vi "1.TCP客户端接收JPEG图片流.vi"() -> ()   [LabVIEW 2018]
panel:
  in  "停止":bool
  out "new picture":picture
  out "接收字符串":string
  out "开始flag":bool=TRUE
  in  "?":string="8088"
  in  "地址输入端":string="192.168.1.30"
  # "地   址："
  # "端口号："
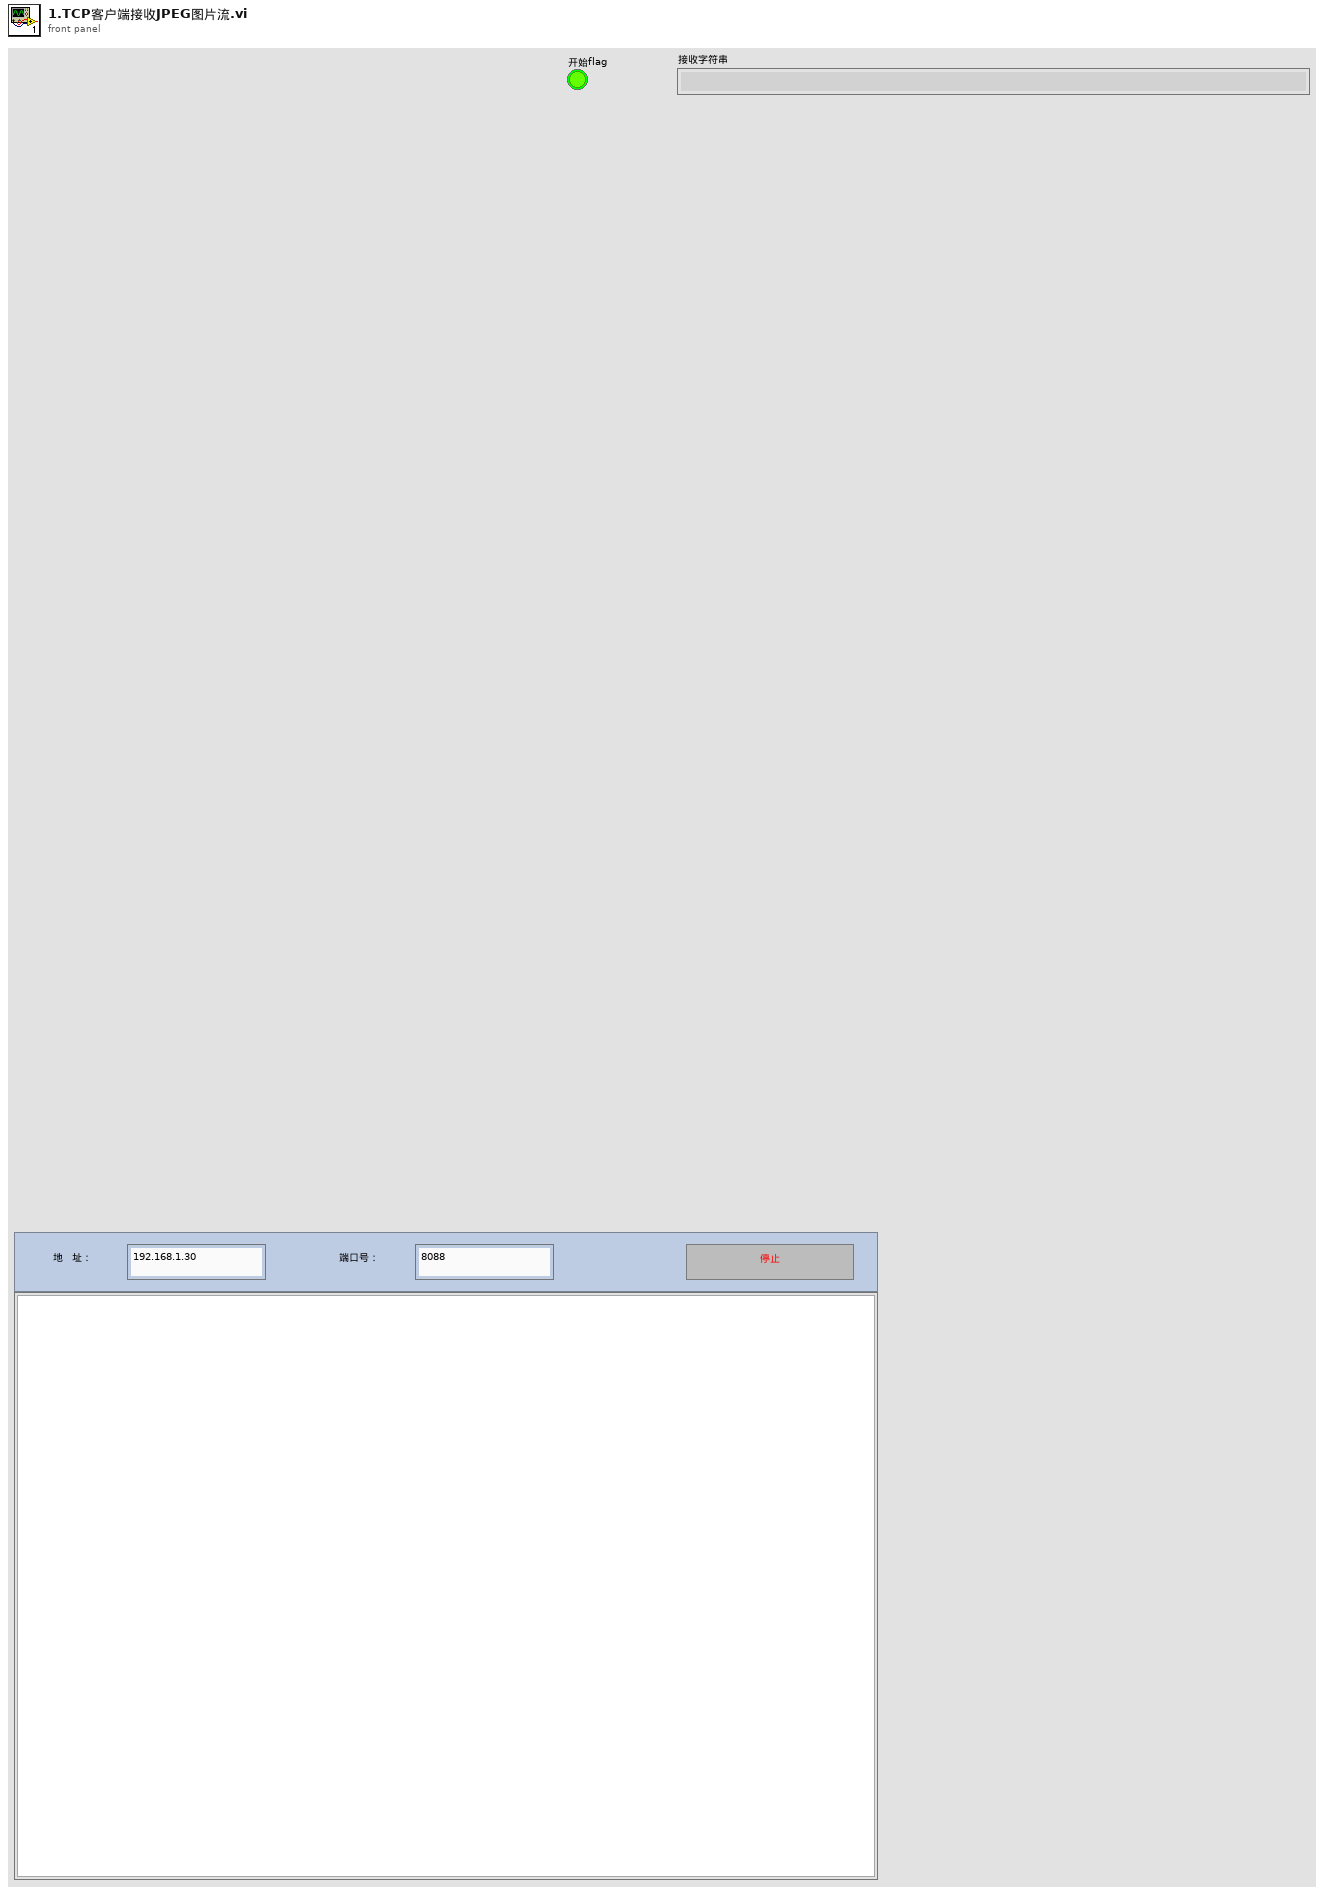
[diagram p1: front panel]
types:
  T1 = enum16{"open", "replace", "create", "open or create", "replace or create", "replace or create with confirmation"}
  T2 = typedef "imagedata.ctl" = cluster{"image type":i32, "image depth":i32, "image":u8[], "mask":u8[], "colors":u32[], "Rectangle":cluster{"left":i16, "top":i16, "right":i16, "bottom":i16}}
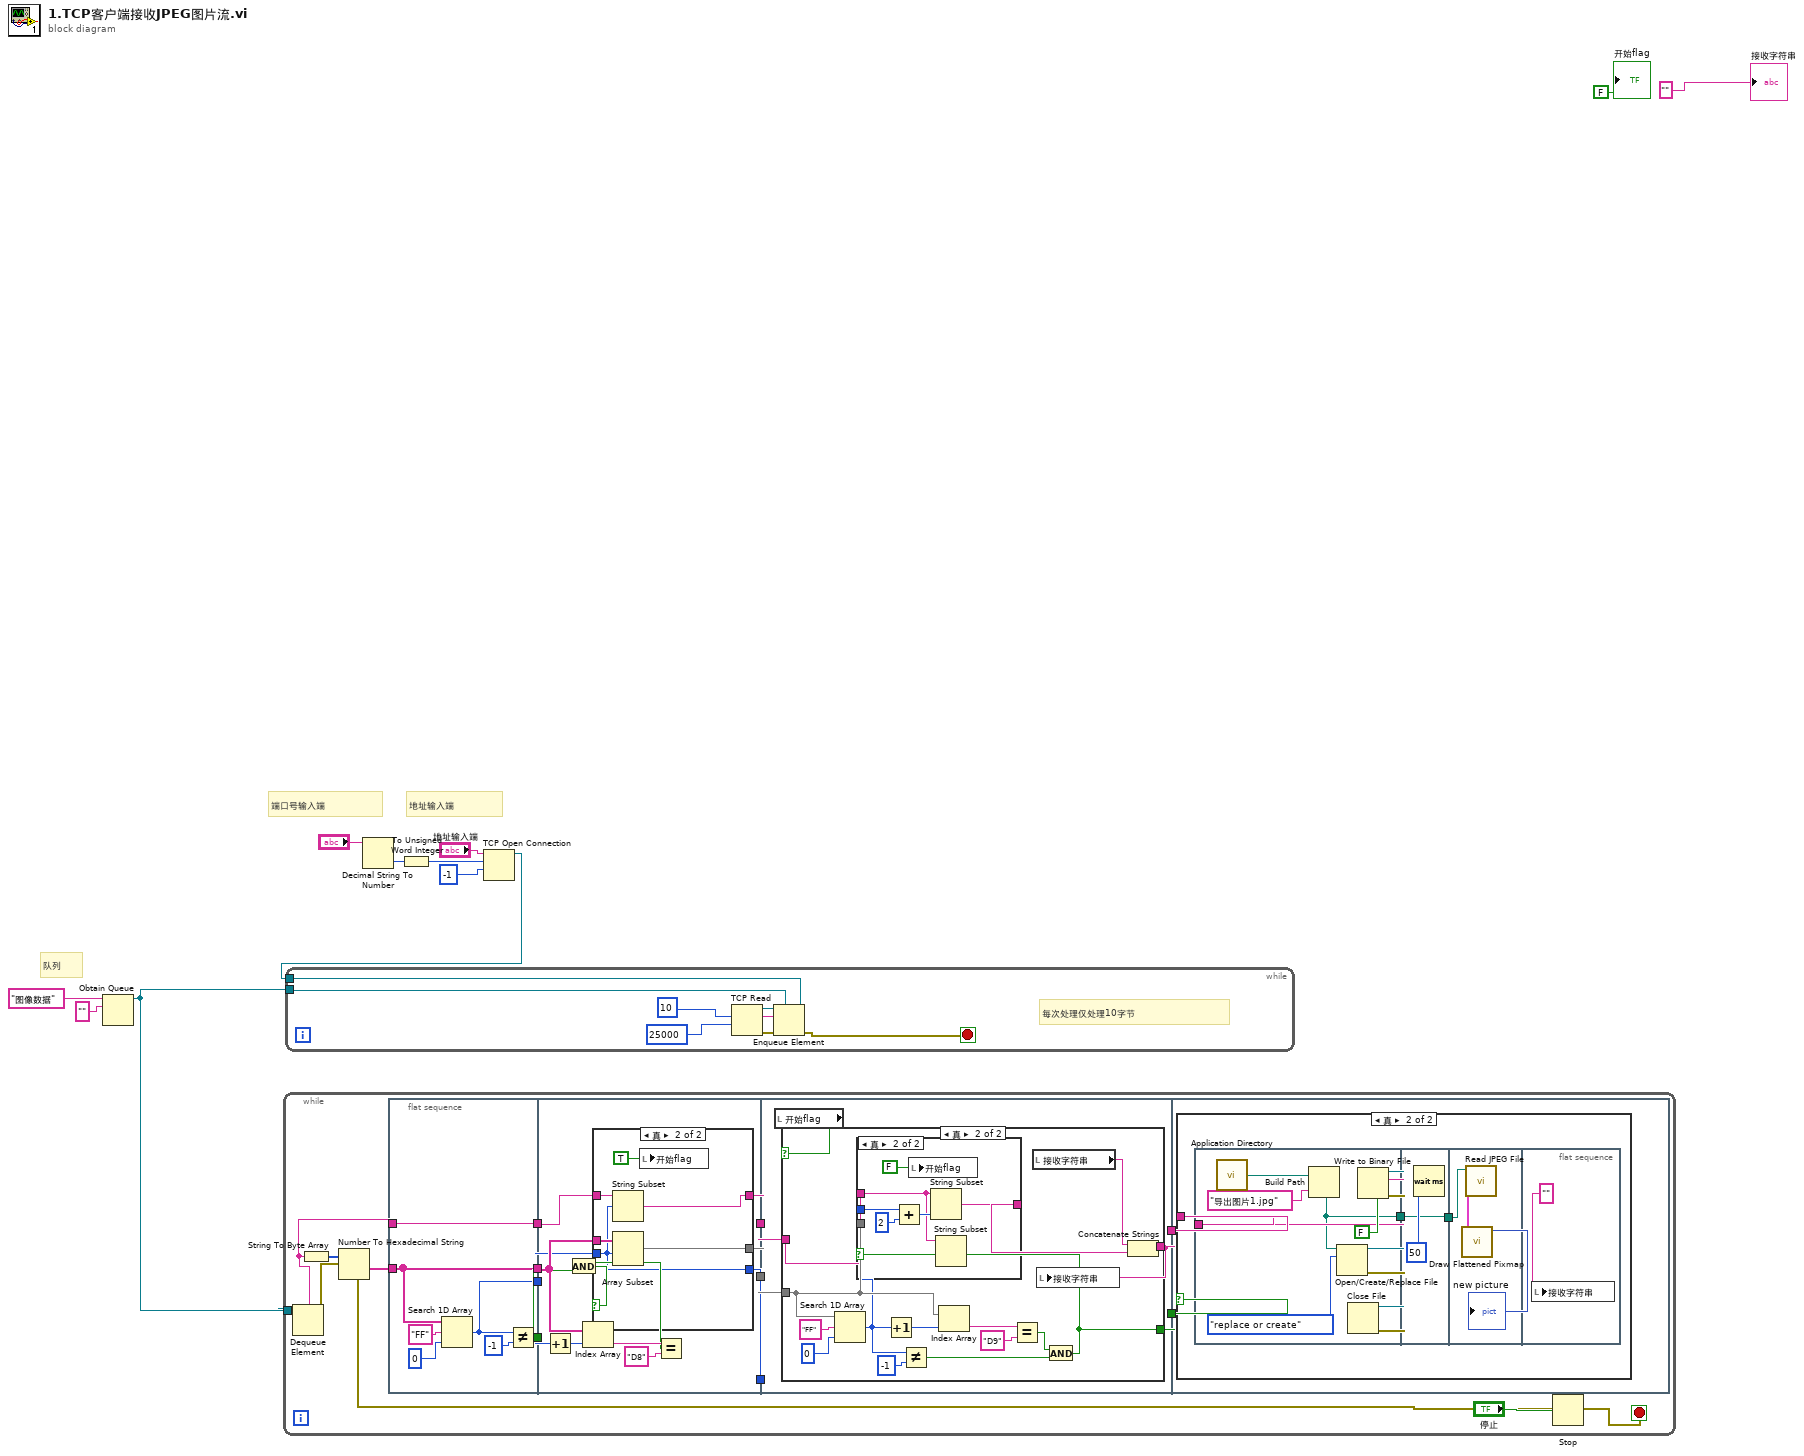
[diagram p0: block diagram]
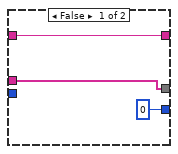
[diagram p2: hidden frame]
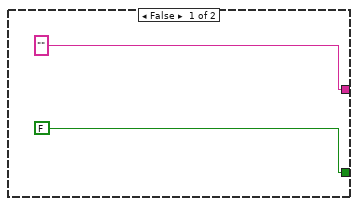
[diagram p3: hidden frame]
diagram:
  # "队列"
  # "端口号输入端"
  # "地址输入端"
  n1 = Obtain Queue(name (unnamed)="图像数据" ("名称（未命名）"), element data type="") -> (queue out=w1:refnum<queue>)  [unwired: 3 in, 2 out]
  n2 = while {
    tunnel: w1 -> [w26]
    stop <- w12 stop-if-true
    n3 = Dequeue Element(queue=w26) -> (element=w14:string, error out=w12:errorcluster)  [unwired: 2 in, 2 out]
    n4 = String To Byte Array(string=w14) -> (unsigned byte array=w15:u8[])
    n5 = Number To Hexadecimal String(2:w15) -> (0:w16:string[])  [unwired: 1 in]
    n6 = flat-sequence {
      tunnel: w16 -> [w32]
      tunnel: [w29] -> w25
      tunnel: [w32] -> w24
      tunnel: w14 -> [w30]
      tunnel: [w30] -> w23
      tunnel: [w27] -> w22
      tunnel: w25 -> [w40]
      tunnel: w24 -> [w44]
      tunnel: [w43] -> w21
      tunnel: [w39] -> w20
      tunnel: w23 -> [w38]
      tunnel: [w37] -> w19
      tunnel: w22 -> [w35]
      tunnel: w21 -> [_]
      tunnel: w20 -> [w58]
      tunnel: w19 -> [w57]
      tunnel: [w56] -> w18
      tunnel: [w55] -> w17
      tunnel: w18 -> [w85]
      tunnel: w17 -> [w84]
      frame #0 {
        n7 = Search 1D Array(1D array=w32, element="FF" ("元素"), start index (0)=0 ("开始索引(0)")) -> (index of element=w29:i32)
        n8 = Not Equal?(x=w29, y=-1) -> (x != y?=w27:bool)
      }
      frame #1 {
        n9 = Increment(x=w40) -> (x+1=w42:i32)
        n10 = Index Array(array=w44, index=w42) -> (element=w45:string)
        n11 = Equal?(x=w45, y="D8") -> (x = y?=w36:bool)
        n12 = And(x=w36, y=w35) -> (x .and. y?=w34:bool)
        n13 = case shown="真" w34 {
          tunnel: w44 -> [w47 w53]
          tunnel: [0 w49] -> w43
          tunnel: w40 -> [_ w49]
          tunnel: [w47 w52] -> w39
          tunnel: [w46 w50] -> w37
          tunnel: w38 -> [w46 w51]
          frame False {
          }
          frame True {
            n14 = String Subset(string=w51, offset (0)=w49) -> (substring=w50:string)  [unwired: 1 in]
            n15 = Array Subset(array=w53, index=w49) -> (w52:string[])  [unwired: 1 in]
            n16 = local write "开始flag"(TRUE ("开始flag")) -> ()
          }
        }
      }
      frame #2 {
        n17 = local read "开始flag"() -> (w59:bool)
        n18 = case shown="真" w59 {
          tunnel: w58 -> [_ w71]
          tunnel: w57 -> [_ w69]
          tunnel: [FALSE w63] -> w56
          tunnel: ["" w62] -> w55
          frame False {
          }
          frame True {
            n19 = Search 1D Array(1D array=w71, element="FF" ("元素"), start index (0)=0 ("开始索引(0)")) -> (index of element=w67:i32)
            n20 = Increment(x=w67) -> (x+1=w74:i32)
            n21 = Not Equal?(x=w67, y=-1) -> (x != y?=w64:bool)
            n22 = Index Array(array=w71, index=w74) -> (element=w72:string)
            n23 = Equal?(x=w72, y="D9") -> (x = y?=w65:bool)
            n24 = local read "接收字符串"() -> (w70:string)
            n25 = And(x=w65, y=w64) -> (x .and. y?=w63:bool)
            n26 = case shown="真" w63 {
              tunnel: w71 -> [_ _]
              tunnel: w67 -> [_ w81]
              tunnel: w69 -> [w77 w78]
              tunnel: [w77 w80] -> w68
              frame False {
              }
              frame True {
                n27 = Add(x=w81, y=2) -> (x+y=w79:i32)
                n28 = local write "开始flag"(FALSE ("开始flag")) -> ()
                n29 = String Subset(string=w78, length (rest)=w79) -> (substring=w80:string)  [unwired: 1 in]
                n30 = String Subset(string=w78) -> ()  [unwired: 2 in, 1 out]
              }
            }
            n31 = Concatenate Strings(w70, w68) -> (w62:string)
            n32 = local write "接收字符串"(w62) -> ()
          }
        }
      }
      frame #3 {
        n33 = case shown="真" w85 {
          tunnel: w84 -> [_ w88]
          frame False {
          }
          frame True {
            n34 = flat-sequence {
              tunnel: w88 -> [w90]
              tunnel: [w89] -> w86
              tunnel: [w99] -> w87
              tunnel: w86 -> [w99]
              tunnel: w87 -> [w101]
              frame #0 {
                n35 = call <vilib>:"Application Directory.vi"() -> ("Application Directory"=w92:path)
                n36 = Build Path(base path=w92, name or relative path="导出图片1.jpg" ("名称或相对路径")) -> (appended path=w89:path)
                n37 = Open/Create/Replace File(file path (use dialog)=w89, operation (0:open)=T1."replace or create" ("操作(0:open)")) -> (refnum out=w93:refnum<file>, error out=w94:errorcluster)  [unwired: 4 in, 1 out]
                n38 = Write to Binary File(file (use dialog)=w93, data=w90, error in=w94, 5:FALSE ("预置数组或字符串大小？(T)")) -> (refnum out=w95:refnum<file>, error out=w96:errorcluster)  [unwired: 2 in, 1 out]
                n39 = Close File(refnum=w95, error in=w96) -> ()  [unwired: 2 out]
              }
              frame #1 {
                n40 = Wait (ms)(milliseconds to wait=u32 50 ("等待时间（毫秒）")) -> ()  [unwired: 1 out]
              }
              frame #2 {
                n41 = call <vilib>:"Read JPEG File.vi"("path to JPEG file"=w101) -> ("image data"=w103:T2)  [unwired: 8 in, 2 out]
                n42 = call <vilib>:"Draw Flattened Pixmap.vi"("image data"=w103) -> ("new picture"=→"new picture":picture)  [unwired: 8 in]
              }
              frame #3 {
                n43 = local write "接收字符串"("") -> ()
              }
            }
          }
        }
      }
    }
    n44 = Stop(stop? (T)="停止") -> ()
  }
  n45 = Decimal String To Number(string="?") -> (number=w7:i32)  [unwired: 2 in, 1 out]
  n46 = To Unsigned Word Integer(number=w7) -> (unsigned 16bit integer=w6:u16)
  n47 = TCP Open Connection(address="地址输入端", remote port or service name=w6, timeout ms (60000)=-1 ("超时毫秒(60000)")) -> (connection ID=w3:refnum<k5>)  [unwired: 2 in, 1 out]
  n48 = while {
    tunnel: w3 -> [w110]
    tunnel: w1 -> [w109]
    stop <- w107 stop-if-true
    # "每次处理仅处理10字节"
    n49 = TCP Read(connection ID=w110, bytes to read=10 ("读取的字节"), 9:25000 ("超时毫秒(25000)")) -> (data out=w108:string, error out=w105:errorcluster)  [unwired: 2 in, 1 out]
    n50 = Enqueue Element(queue=w109, element=w108, error in (no error)=w105) -> (error out=w107:errorcluster)  [unwired: 1 in, 2 out]
  }
  "开始flag" <- FALSE ("布尔")
  "接收字符串" <- ""
